vi "Update_1layer_Wx_with_FPGA.vi"(2 "error in (no error)":errorcluster, 3 "FPGA VI Reference In":refnum<k20>, 5 "Learning rate":fxp<+/-,32,8>, 6 "1layer_Out_hx":fxp<+/-,32,8>, 7 "Array_Weights_hx":fxp<+/-,32,8>[](array[numeric]), 8 "Array_Inputs":fxp<+/-,32,8>[](array[numeric]), 9 "Array_2layer_Weights_at_Index_hx":fxp<+/-,32,8>[](array[numeric]), 10 "Array_Out_ox":fxp<+/-,32,8>[](array[numeric]), 11 "Array_target_ox":fxp<+/-,32,8>[](array[numeric])) -> (0 "FPGA VI Reference Out":refnum<k20>, 1 "error out":errorcluster, 4 "Array_Weights_hx_updated":fxp<+/-,32,8>[](array[numeric]))   [LabVIEW 2016]
uses:
  <vilib>/Utility/error.llb/Error Cluster From Error Code.vi
  <vilib>/rvi/errors/niLvFpgaAdjustHostInterfaceError.vi
  <vilib>/rvi/interface/nirviReadWriteControl/nirviReadWriteControl.xnode
  NiFpgaLv.dll
  <vilib>/rvi/interface/Simulation/niFpgaSimulationCallBeginRW.vi
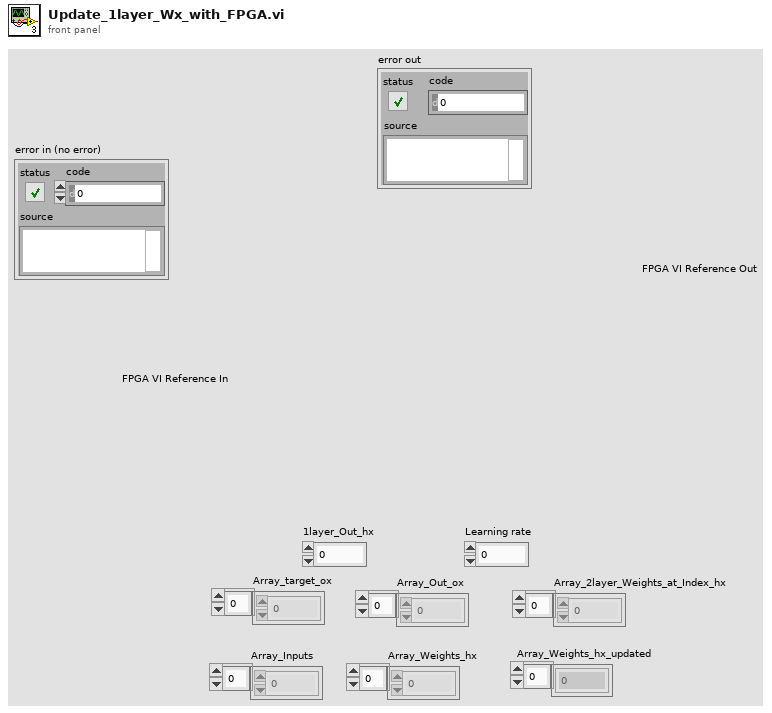
[diagram p1: front panel]
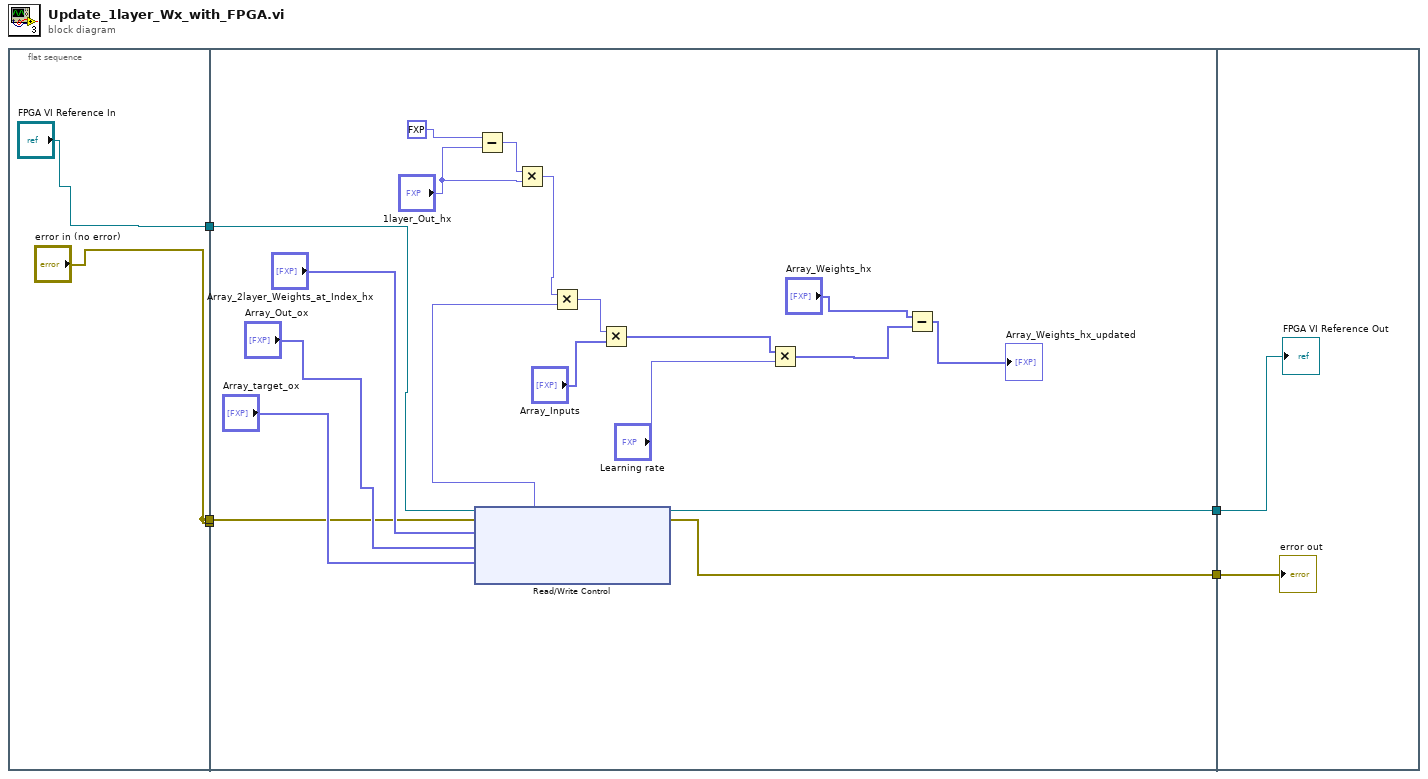
[diagram p0: block diagram]
diagram:
  n1 = flat-sequence {
    tunnel: ["FPGA VI Reference In"] -> w5
    tunnel: ["error in (no error)"] -> w2
    tunnel: ["error in (no error)"] -> w1
    tunnel: w5 -> [w15]
    tunnel: [w10] -> w4
    tunnel: [w9] -> w3
    tunnel: w2 -> [_]
    tunnel: w1 -> [w8]
    tunnel: w4 -> [w28]
    tunnel: w3 -> [w27]
    frame #0 {
    }
    frame #1 {
      n2 = xnode "Read/Write Control"("FPGA VI Reference In"=w15, "error in"=w8, "Array_2layer_Weights_at_Index_hx"="Array_2layer_Weights_at_Index_hx", "Array_Out_ox"="Array_Out_ox", "Array_target_ox"="Array_target_ox") -> ("FPGA VI Reference Out"=w10:refnum<k20>, "error out"=w9:errorcluster, "Err_outX"=w14:fxp<+/-,32,8>)
      n3 = Subtract(x=fxp<+,32,8> 1.0, y="1layer_Out_hx") -> (x-y=w18:fxp<+/-,34,10>)
      n4 = Multiply(x=w18, y="1layer_Out_hx") -> (x*y=w16:fxp<+/-,32,8>)
      n5 = Multiply(x=w16, y=w14) -> (x*y=w24:fxp<+/-,32,8>)
      n6 = Multiply(x=w24, y="Array_Inputs") -> (x*y=w22:fxp<+/-,32,8>[])
      n7 = Multiply(x=w22, y="Learning rate") -> (x*y=w20:fxp<+/-,32,8>[])
      n8 = Subtract(x="Array_Weights_hx", y=w20) -> (x-y=→"Array_Weights_hx_updated":fxp<+/-,32,8>[])
    }
    frame #2 {
      "error out" <- w27
      "FPGA VI Reference Out" <- w28
    }
  }
